vi "Check CCD_CF.vi"(8 "error in (no error)":errorcluster, 10 "Resp ACS":string, 11 "Interface in":refnum<class "Interface.lvclass">) -> (0 "error out":errorcluster, 3 "Interface out":refnum<class "Interface.lvclass">)   [LabVIEW 2018, in "Interface.lvclass"]
uses:
  Interface.lvclass
  Interface.lvclass/Interface.ctl
panel:
  in  "value":T1
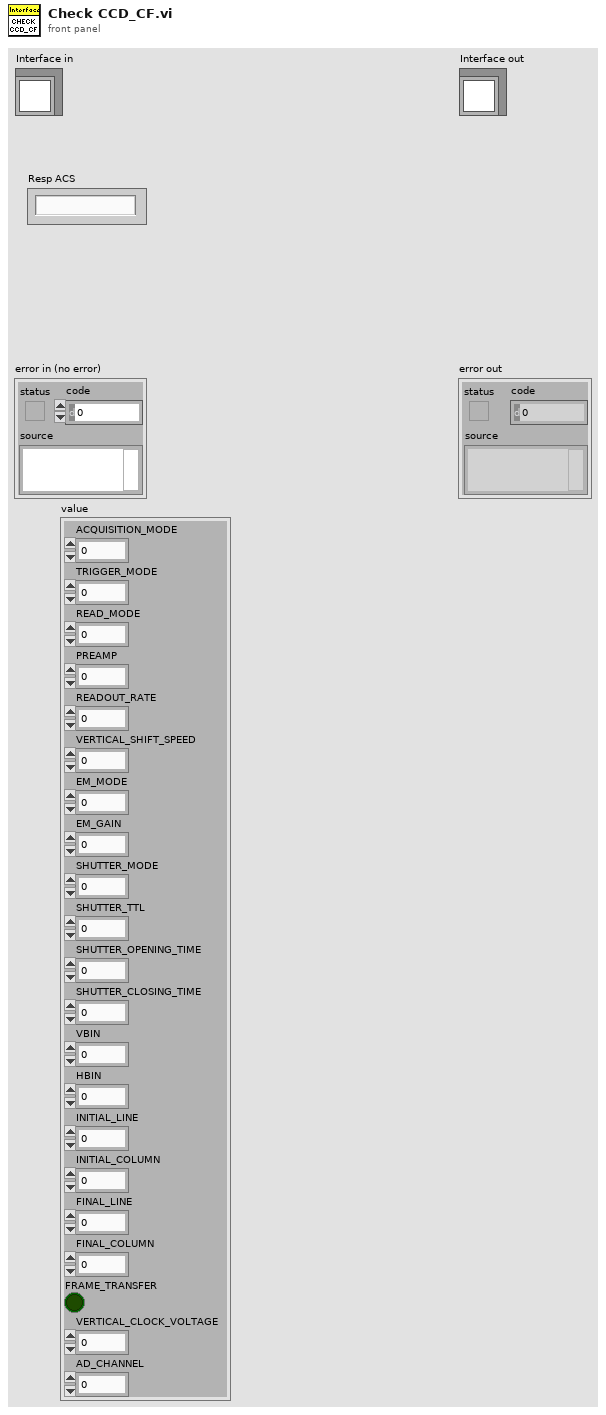
[diagram p1: front panel]
types:
  T1 = cluster{"ACQUISITION_MODE":u8, "TRIGGER_MODE":u8, "READ_MODE":u8, "PREAMP":u8, "READOUT_RATE":u8, "VERTICAL_SHIFT_SPEED":u8, "EM_MODE":u8, "EM_GAIN":u16, "SHUTTER_MODE":u8, "SHUTTER_TTL":u8, "SHUTTER_OPENING_TIME":u16, "SHUTTER_CLOSING_TIME":u16, "VBIN":u16, "HBIN":u16, "INITIAL_LINE":u16, "INITIAL_COLUMN":u16, "FINAL_LINE":u16, "FINAL_COLUMN":u16, "FRAME_TRANSFER":bool, "VERTICAL_CLOCK_VOLTAGE":u8, "AD_CHANNEL":u32}
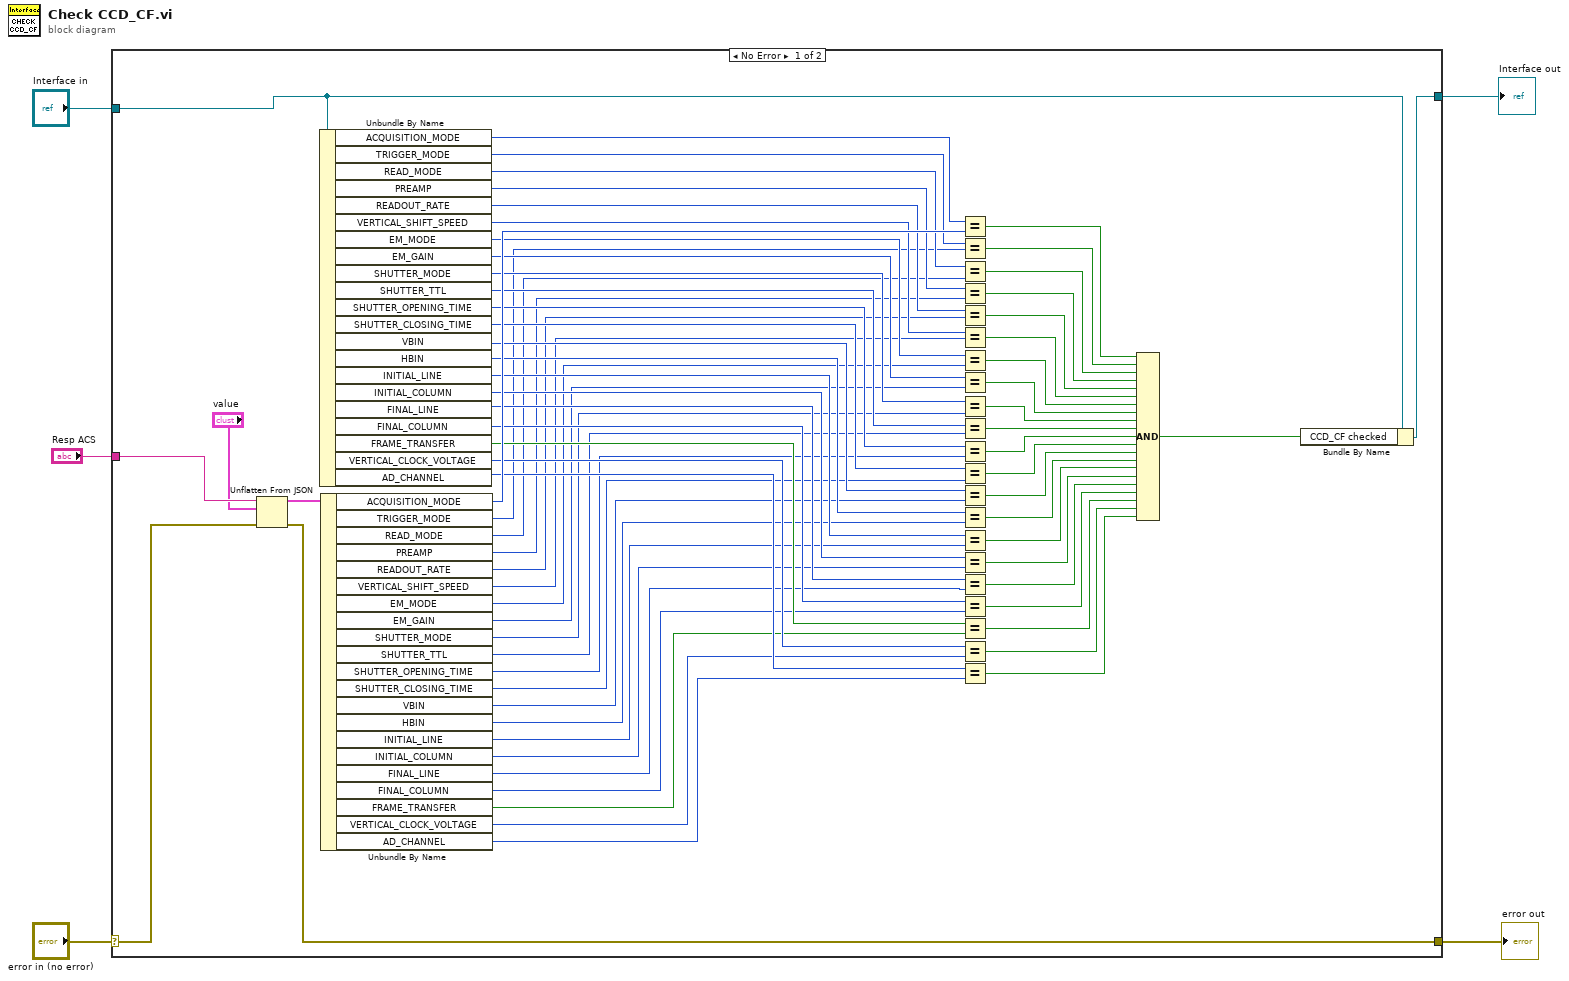
[diagram p0: block diagram]
diagram:
  n1 = case shown="No Error" "error in (no error)" {
    selector: "error in (no error)" -> [w8 w78]
    tunnel: [w9 w78] -> w4
    tunnel: [w12 w77] -> w2
    tunnel: "Interface in" -> [w7 w77]
    tunnel: "Resp ACS" -> [w76 _]
    frame No Error {
      n2 = Unflatten From JSON(JSON string=w76, type and defaults="value", error in (no error)=w8) -> (value=w11:T1, error out=w9:errorcluster)  [unwired: 4 in]
      n3 = Unbundle By Name(w7) -> ("ACQUISITION_MODE"=w75:u8, "TRIGGER_MODE"=w73:u8, "READ_MODE"=w72:u8, "PREAMP"=w71:u8, "READOUT_RATE"=w70:u8, "VERTICAL_SHIFT_SPEED"=w69:u8, "EM_MODE"=w68:u8, "EM_GAIN"=w67:u16, "SHUTTER_MODE"=w66:u8, "SHUTTER_TTL"=w65:u8, "SHUTTER_OPENING_TIME"=w64:i32, "SHUTTER_CLOSING_TIME"=w63:i32, "VBIN"=w62:u16, "HBIN"=w61:u16, "INITIAL_LINE"=w60:u16, "INITIAL_COLUMN"=w59:u16, "FINAL_LINE"=w58:u16, "FINAL_COLUMN"=w57:u16, "FRAME_TRANSFER"=w56:bool, "VERTICAL_CLOCK_VOLTAGE"=w55:u8, "AD_CHANNEL"=w54:u32)
      n4 = Unbundle By Name(w11) -> ("ACQUISITION_MODE"=w74:u8, "TRIGGER_MODE"=w53:u8, "READ_MODE"=w52:u8, "PREAMP"=w51:u8, "READOUT_RATE"=w50:u8, "VERTICAL_SHIFT_SPEED"=w49:u8, "EM_MODE"=w48:u8, "EM_GAIN"=w47:u16, "SHUTTER_MODE"=w46:u8, "SHUTTER_TTL"=w45:u8, "SHUTTER_OPENING_TIME"=w44:u16, "SHUTTER_CLOSING_TIME"=w43:u16, "VBIN"=w42:u16, "HBIN"=w41:u16, "INITIAL_LINE"=w40:u16, "INITIAL_COLUMN"=w39:u16, "FINAL_LINE"=w38:u16, "FINAL_COLUMN"=w37:u16, "FRAME_TRANSFER"=w36:bool, "VERTICAL_CLOCK_VOLTAGE"=w35:u8, "AD_CHANNEL"=w34:u32)
      n5 = Equal?(x=w75, y=w74) -> (x = y?=w33:bool)
      n6 = Equal?(x=w73, y=w53) -> (x = y?=w32:bool)
      n7 = Equal?(x=w72, y=w52) -> (x = y?=w31:bool)
      n8 = Equal?(x=w71, y=w51) -> (x = y?=w30:bool)
      n9 = Equal?(x=w70, y=w50) -> (x = y?=w29:bool)
      n10 = Equal?(x=w69, y=w49) -> (x = y?=w28:bool)
      n11 = Equal?(x=w68, y=w48) -> (x = y?=w27:bool)
      n12 = Equal?(x=w67, y=w47) -> (x = y?=w26:bool)
      n13 = Equal?(x=w66, y=w46) -> (x = y?=w25:bool)
      n14 = Equal?(x=w65, y=w45) -> (x = y?=w24:bool)
      n15 = Equal?(x=w64, y=w44) -> (x = y?=w23:bool)
      n16 = Equal?(x=w63, y=w43) -> (x = y?=w22:bool)
      n17 = Equal?(x=w62, y=w42) -> (x = y?=w21:bool)
      n18 = Equal?(x=w61, y=w41) -> (x = y?=w20:bool)
      n19 = Equal?(x=w60, y=w40) -> (x = y?=w19:bool)
      n20 = Equal?(x=w59, y=w39) -> (x = y?=w18:bool)
      n21 = Equal?(x=w58, y=w38) -> (x = y?=w17:bool)
      n22 = Equal?(x=w57, y=w37) -> (x = y?=w16:bool)
      n23 = Equal?(x=w56, y=w36) -> (x = y?=w15:bool)
      n24 = Equal?(x=w55, y=w35) -> (x = y?=w14:bool)
      n25 = Equal?(x=w54, y=w34) -> (x = y?=w13:bool)
      n26 = Compound Arithmetic op=AND(w33, w32, w31, w30, w29, w28, w27, w26, w25, w24, w23, w22, w21, w20, w19, w18, w17, w16, w15, w14, w13) -> (w10:bool)
      n27 = Bundle By Name(cluster=w7, "CCD_CF checked"=w10) -> (w12:refnum<class "Interface.lvclass">)
    }
    frame Error {
    }
  }
  "error out" <- w4
  "Interface out" <- w2
